vi "Light Intensity.vi"(7 "Get/Set":enum16{"Get", "Set"}(ring), 8 "error in (no error)":errorcluster, 9 "Intensity In":dbl, 10 "Light Name":string, 11 "FlexWorktable in":refnum<class "FlexWorktable.lvclass">) -> (0 "error out":errorcluster, 1 "Intensity out":dbl, 3 "FlexWorktable out":refnum<class "FlexWorktable.lvclass">)   [LabVIEW 2017, in "FlexWorktable.lvclass"]
uses:
  FlexWorktable.lvclass
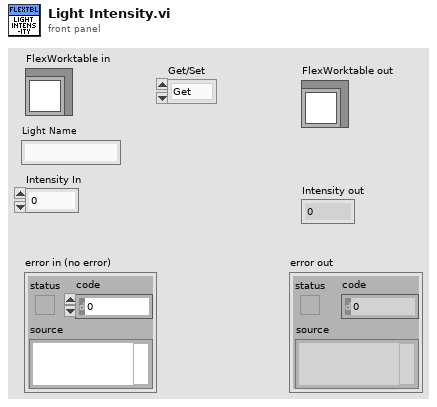
[diagram p1: front panel]
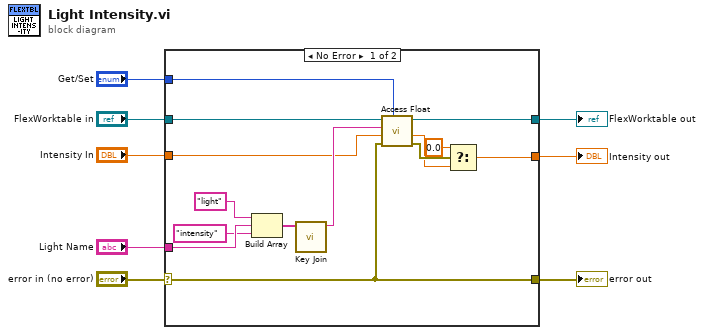
[diagram p0: block diagram]
diagram:
  n1 = case shown="No Error" "error in (no error)" {
    selector: "error in (no error)" -> [w9 w25]
    tunnel: [w9 w25] -> w7
    tunnel: [w11 w24] -> w5
    tunnel: "FlexWorktable in" -> [w22 w24]
    tunnel: "Light Name" -> [w19 _]
    tunnel: "Get/Set" -> [w16 _]
    tunnel: "Intensity In" -> [w15 w23]
    tunnel: [w10 w23] -> w1
    frame No Error {
      n2 = Build Array("light" ("element"), w19, "intensity" ("element")) -> (w21:string[])
      n3 = call "Key Join.vi"("Key Elements"=w21) -> ("Key"=w20:string)  [unwired: 10 in]
      n4 = call-dynamic "Access Float.vi"("Get/Set"=w16, "error in (no error)"=w9, "Value in"=w15, "Key"=w20, "FlexWorktable in"=w22) -> ("error out"=w14:errorcluster, "Value out"=w13:dbl, "FlexWorktable out"=w11:refnum<class "FlexWorktable.lvclass">)  [unwired: 4 in]
      n5 = Select(t=0.0, s=w14, f=w13) -> (s? t:f=w10:dbl)
    }
    frame Error {
    }
  }
  "error out" <- w7
  "FlexWorktable out" <- w5
  "Intensity out" <- w1
